vi "test-linear-quadratic-regulator.vi"(8 "error in (no error)":errorcluster) -> (0 "error out":errorcluster, 3 "ALL TESTS GOOD":bool)   [LabVIEW 2019]
uses:
  <vilib>/Rock Robotics/WPI/ThirdParty/JAS_Junk/TrajLib/LINEAR_SYSTEM.ctl
  <vilib>/Analysis/Matrix/Datatypes/RealMatrix.ctl
  <vilib>/Rock Robotics/WPI/ThirdParty/JAS_Junk/TrajLib/LINEAR_QUADRATIC_REGULATOR.ctl
  <vilib>/Rock Robotics/WPI/ThirdParty/JAS_Junk/TrajLib/MatBuilder_Create.vi
  <vilib>/Rock Robotics/WPI/ThirdParty/JAS_Junk/TrajLib/DCMotor_New.vi
  <vilib>/Rock Robotics/WPI/ThirdParty/JAS_Junk/TrajLib/Units_RotationsPerMinuteToRadiansPerSecond.vi
  <vilib>/Rock Robotics/WPI/ThirdParty/JAS_Junk/TrajLib/MatrixHelper_Zero.vi
  <vilib>/Rock Robotics/WPI/ThirdParty/JAS_Junk/TrajLib/LinearSystem_New.vi
  <vilib>/Rock Robotics/WPI/ThirdParty/JAS_Junk/TrajLib/Trajectory_Library.lvlib
  <vilib>/Analysis/Matrix/NI_Matrix.lvlib
panel:
  out "Test 5 Good":bool
  out "Test 4-1 Good":bool
  out "Test 2 Good":bool
  out "Test 1 Good":bool
  out "K 5":T1
  out "Error 5":bool
  out "LinearQuadraticRegulator 5":T2
  out "Relms 5":T1
  out "Qelms 5":T1
  out "ElevatorSystem 5":T3
  out "K 4":T1
  out "ExponentNotRational 4-1":bool
  out "Error 4-1":bool
  out "Error 4":bool
  out "K 4-1":T1
  out "LinearQuadraticRegulator 4":T2
  out "Relms 4":T1
  out "Qelms 4":T1
  out "ElevatorSystem 4":T3
  out "Error 2":bool
  out "K 2":T1
  out "LinearQuadraticRegulator 2":T2
  out "Relms 2":T1
  out "Qelms 2":T1
  out "ElevatorSystem 2":T3
  out "K 1":T1
  out "Error 1":bool
  out "Relms 1":T1
  out "Qelms 1":T1
  out "LQR New Sys-ELMS 1":T2
  out "ElevatorSystem 1":T3
  # "assertEquals(522.153, k.get(0, 0), 0.1);\n    assertEquals(38.2, k.get(0, 1), 0.1);"
  # "assertEquals(10.381, regulator.getK().get(0, 0), 1e-2);\n    assertEquals(0.6929, regulator.getK().get(0, 1), 1e-2);"
  # "assertEquals(8.97115941, regulator.getK().get(0, 0), 1e-3);\n    assertEquals(0.07904881, regulator.getK().get(0, 1), 1e-3);"
  # "assertEquals(19.16, k.get(0, 0), 0.1);\n    assertEquals(3.32, k.get(0, 1), 0.1);"
  # "Ref State <States,1>"
  # "Comp and capped \noutput <Inputs,1>"
  # "Controller gain\n<Inputs,States>"
  # "<States,States>"
  # "<States,Inputs>"
  # "<Outputs,States>"
  # "<Outputs,Inputs>"
  # "Ref State <States,1>"
  # "Comp and capped \noutput <Inputs,1>"
  # "Controller gain\n<Inputs,States>"
  # "<States,States>"
  # "<States,Inputs>"
  # "<Outputs,States>"
  # "<Outputs,Inputs>"
  # "Ref State <States,1>"
  # "Comp and capped \noutput <Inputs,1>"
  # "Controller gain\n<Inputs,States>"
  # "<States,States>"
  # "<States,Inputs>"
  # "<Outputs,States>"
  # "<Outputs,Inputs>"
  # "Ref State <States,1>"
  # "Comp and capped \noutput <Inputs,1>"
  # "Controller gain\n<Inputs,States>"
  # "<States,States>"
  # "<States,Inputs>"
  # "<Outputs,States>"
  # "<Outputs,Inputs>"
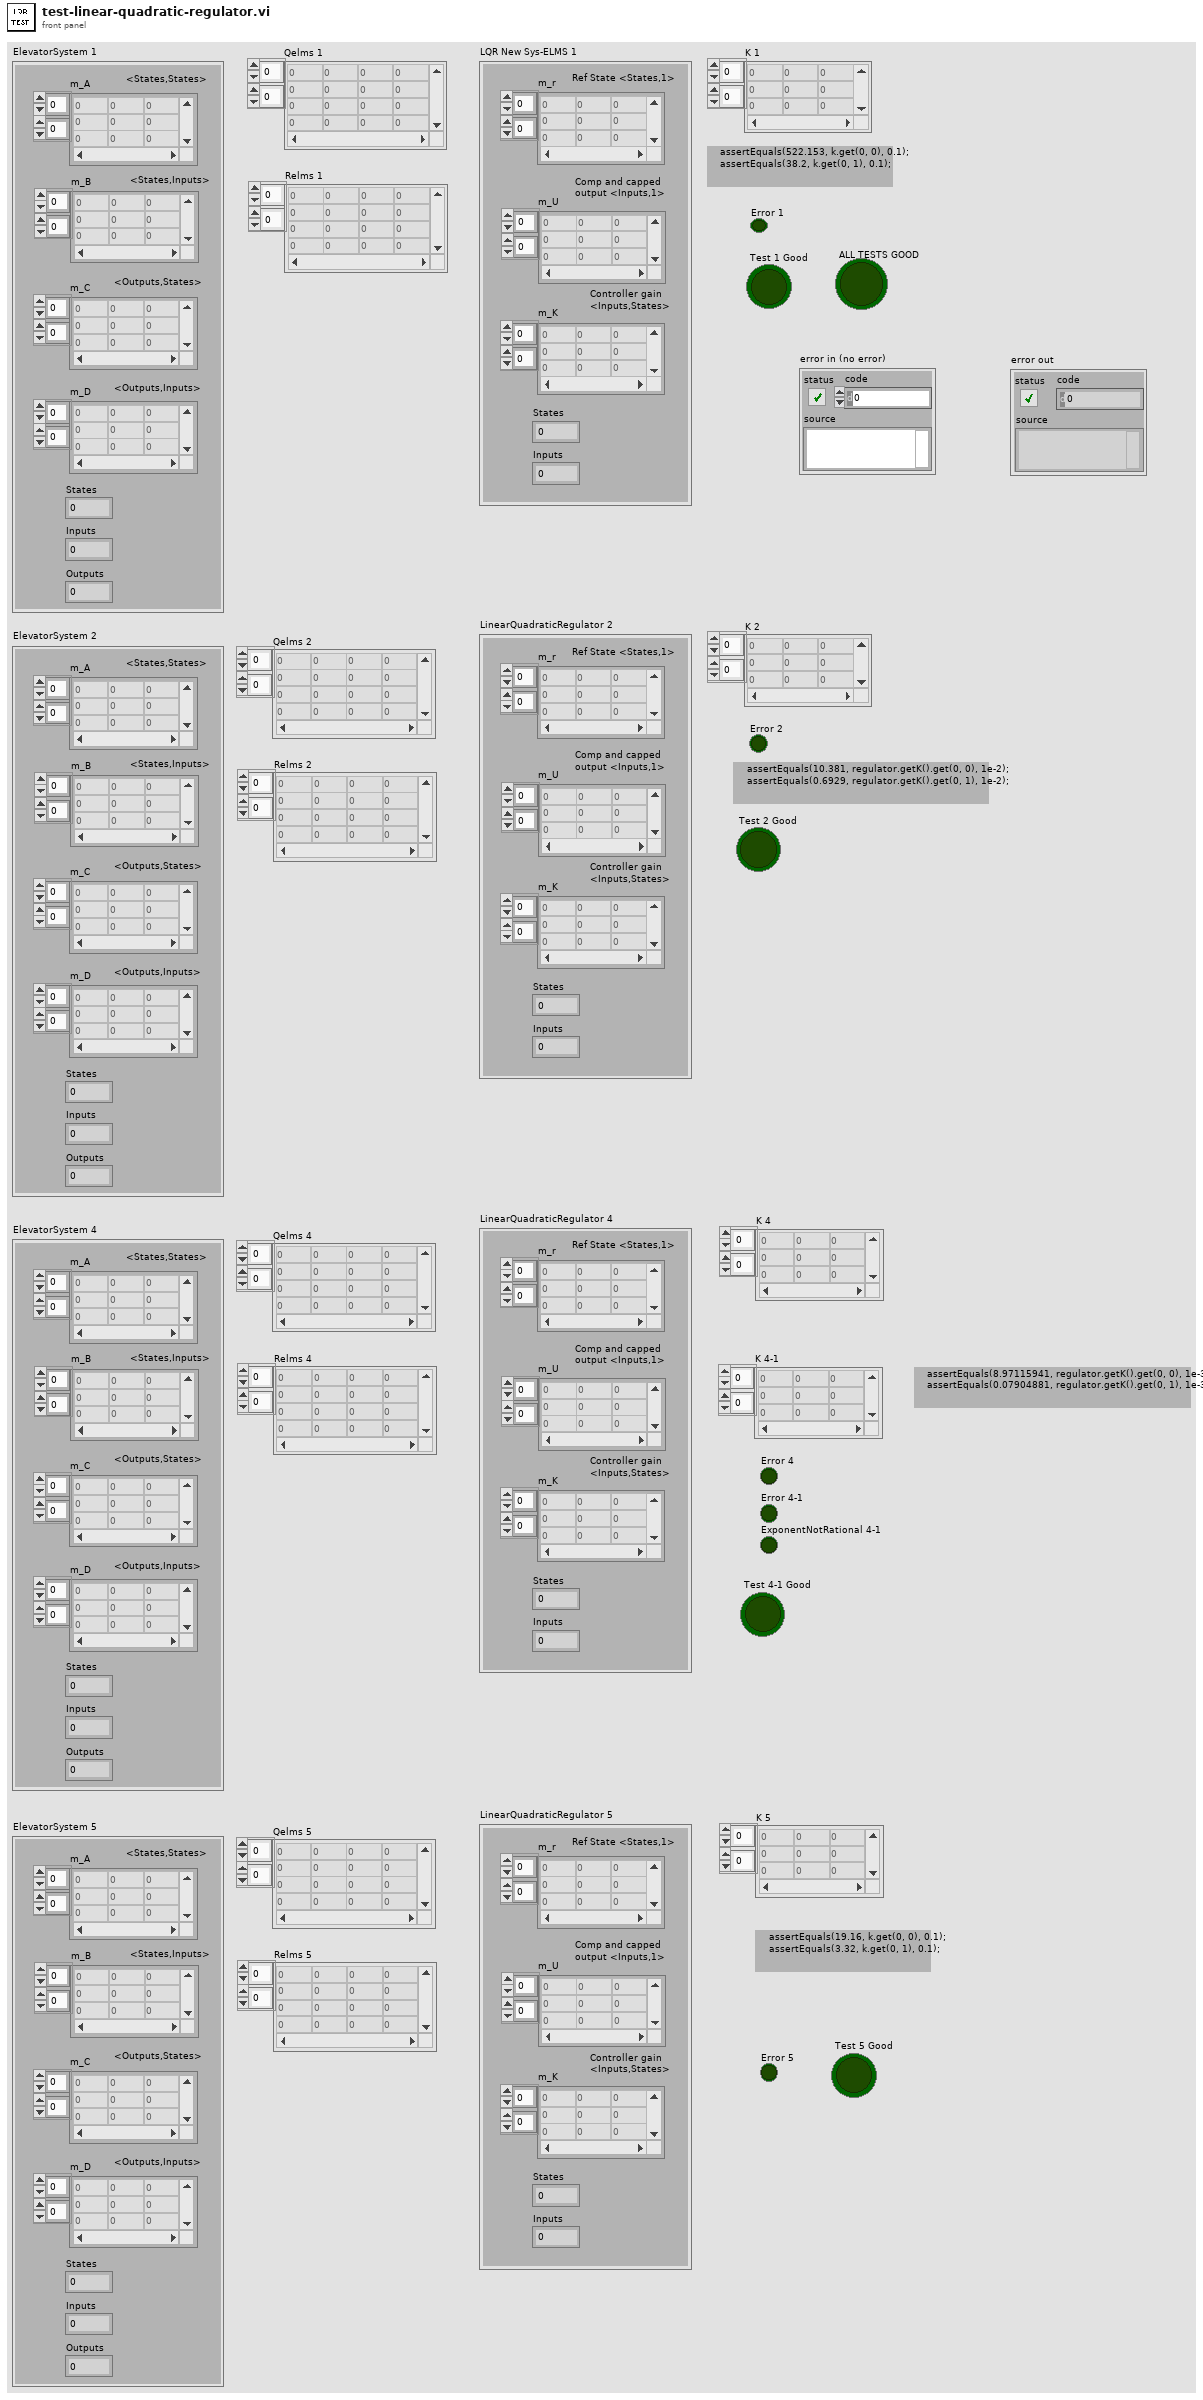
[diagram p1: front panel]
types:
  T1 = typedef "NI_Matrix.lvlib/RealMatrix.ctl" = dbl[][]
  T2 = typedef "Trajectory_Library.lvlib/LINEAR_QUADRATIC_REGULATOR.ctl" = cluster{"m_r":T1, "m_U":T1, "m_K":T1, "States":i32, "Inputs":i32}
  T3 = typedef "Trajectory_Library.lvlib/LINEAR_SYSTEM.ctl" = cluster{"m_A":T1, "m_B":T1, "m_C":T1, "m_D":T1, "States":i32, "Inputs":i32, "Outputs":i32}
  T4 = typedef "Trajectory_Library.lvlib/DCMOTOR.CTL" = cluster{"nominalVoltage_Volts":dbl, "StallTorque_NM":dbl, "StallCurrent_Amps":dbl, "FreeCurrent_Amps":dbl, "FreeSpeed_RadPerSec":dbl, "R_Ohms":dbl, "KvINV_RadPerSecPerVolt":dbl, "Kt_NMPerAmp":dbl, "L_H":dbl, "Jr_KgM2":dbl}
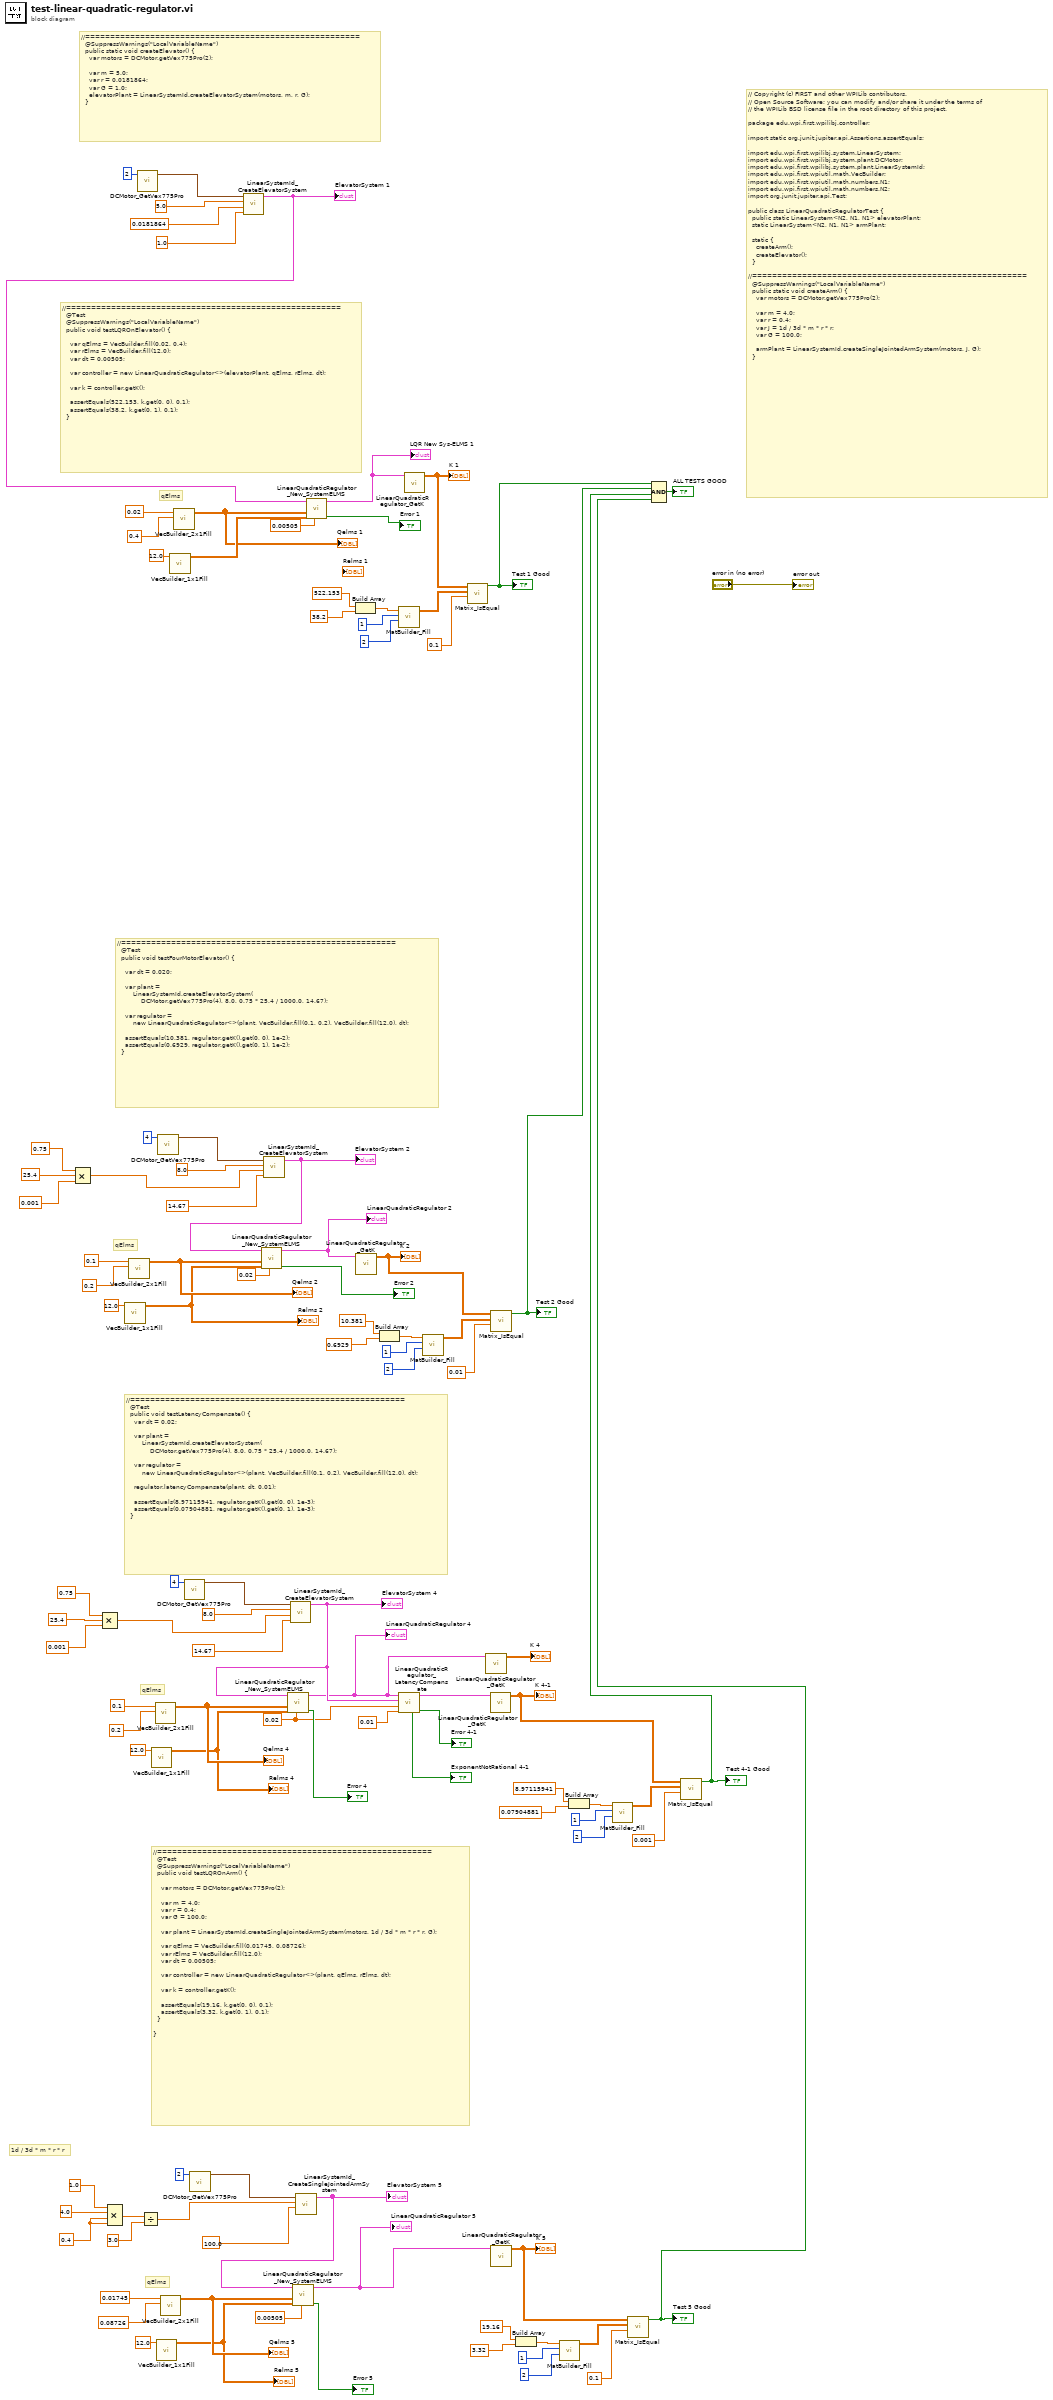
[diagram p0: block diagram]
diagram:
  w43 = 0.4 ("value")
  w63 = 0.02 ("dt_Seconds")
  # "1d / 3d * m * r * r"
  # "qElms"
  # "//=======================================================\n  @Test\n  @SuppressWarnings(\"LocalVariableName\")\n  public void testLQROnArm() {\n\n    var motors = DCMotor.getVex775Pro(2);\n\n    var m = 4.0;\n    var r = 0.4;\n    var G = 100.0;\n\n    var plant = LinearSystemId.createSingleJointedArmSystem(motors, 1d / 3d * m * r * r, G);\n\n    var qElms = VecBuilder.fill(0.01745, 0.08726);\n    var rElms = VecBuilder.fill(12.0);\n    var dt = 0.00505;\n\n    var controller = new LinearQuadraticRegulator<>(plant, qElms, rElms, dt);\n\n    var k = controller.getK();\n\n    assertEquals(19.16, k.get(0, 0), 0.1);\n    assertEquals(3.32, k.get(0, 1), 0.1);\n  }\n\n}"
  # "qElms"
  # "//=======================================================\n  @Test\n  public void testLatencyCompensate() {\n    var dt = 0.02;\n\n    var plant =\n        LinearSystemId.createElevatorSystem(\n            DCMotor.getVex775Pro(4), 8.0, 0.75 * 25.4 / 1000.0, 14.67);\n\n    var regulator =\n        new LinearQuadraticRegulator<>(plant, VecBuilder.fill(0.1, 0.2), VecBuilder.fill(12.0), dt);\n\n    regulator.latencyCompensate(plant, dt, 0.01);\n\n    assertEquals(8.97115941, regulator.getK().get(0, 0), 1e-3);\n    assertEquals(0.07904881, regulator.getK().get(0, 1), 1e-3);\n  }"
  # "qElms"
  # "//=======================================================\n  @Test\n  public void testFourMotorElevator() {\n\n    var dt = 0.020;\n\n    var plant =\n        LinearSystemId.createElevatorSystem(\n            DCMotor.getVex775Pro(4), 8.0, 0.75 * 25.4 / 1000.0, 14.67);\n\n    var regulator =\n        new LinearQuadraticRegulator<>(plant, VecBuilder.fill(0.1, 0.2), VecBuilder.fill(12.0), dt);\n\n    assertEquals(10.381, regulator.getK().get(0, 0), 1e-2);\n    assertEquals(0.6929, regulator.getK().get(0, 1), 1e-2);\n  }"
  # "//=======================================================\n  @SuppressWarnings(\"LocalVariableName\")\n  public static void createElevator() {\n    var motors = DCMotor.getVex775Pro(2);\n\n    var m = 5.0;\n    var r = 0.0181864;\n    var G = 1.0;\n    elevatorPlant = LinearSystemId.createElevatorSystem(motors, m, r, G);\n  }"
  # "qElms"
  # "//=======================================================\n  @Test\n  @SuppressWarnings(\"LocalVariableName\")\n  public void testLQROnElevator() {\n\n    var qElms = VecBuilder.fill(0.02, 0.4);\n    var rElms = VecBuilder.fill(12.0);\n    var dt = 0.00505;\n\n    var controller = new LinearQuadraticRegulator<>(elevatorPlant, qElms, rElms, dt);\n\n    var k = controller.getK();\n\n    assertEquals(522.153, k.get(0, 0), 0.1);\n    assertEquals(38.2, k.get(0, 1), 0.1);\n  }"
  # "// Copyright (c) FIRST and other WPILib contributors.\n// Open Source Software; you can modify and/or share it under the terms of\n// the WPILib BSD license file in the root directory of this project.\n\npackage edu.wpi.first.wpilibj.controller;\n\nimport static org.junit.jupiter.api.Assertions.assertEquals;\n\nimport edu.wpi.first.wpilibj.system.LinearSystem;\nimport edu.wpi.first.wpilibj.system.plant.DCMotor;\nimport edu.wpi.first.wpilibj.system.plant.LinearSystemId;\nimport edu.wpi.first.wpiutil.math.VecBuilder;\nimport edu.wpi.first.wpiutil.math.numbers.N1;\nimport edu.wpi.first.wpiutil.math.numbers.N2;\nimport org.junit.jupiter.api.Test;\n\npublic class LinearQuadraticRegulatorTest {\n  public static LinearSystem<N2, N1, N1> elevatorPlant;\n  static LinearSystem<N2, N1, N1> armPlant;\n\n  static {\n    createArm();\n    createElevator();\n  }\n\n//=======================================================\n  @SuppressWarnings(\"LocalVariableName\")\n  public static void createArm() {\n    var motors = DCMotor.getVex775Pro(2);\n\n    var m = 4.0;\n    var r = 0.4;\n    var J = 1d / 3d * m * r * r;\n    var G = 100.0;\n\n    armPlant = LinearSystemId.createSingleJointedArmSystem(motors, J, G);\n  }"
  n1 = Compound Arithmetic op=MULTIPLY(0.75 ("value"), 25.4 ("value"), 0.001 ("value")) -> (w88:dbl)
  n2 = Compound Arithmetic op=MULTIPLY(0.75 ("value"), 25.4 ("value"), 0.001 ("value")) -> (w71:dbl)
  n3 = Compound Arithmetic op=MULTIPLY(1.0 ("value"), 4.0 ("value"), w43, w43) -> (w42:dbl)
  n4 = call <vilib>:"VecBuilder_1x1Fill.vi"("R0_C0"=12.0) -> ("output matrix"=w81:T1)  [unwired: 10 in]
  "Relms 2" <- w81
  n5 = call <vilib>:"VecBuilder_2x1Fill.vi"("R1"=0.2, "R0"=0.1) -> ("output matrix"=w83:T1)  [unwired: 9 in]
  "Qelms 2" <- w83
  n6 = call <vilib>:"DCMotor_GetVex775Pro.vi"("Num Motors"=2) -> ("DCMOTOR"=w105:T4)  [unwired: 10 in]
  n7 = Divide(x=w42, y=3.0) -> (x/y=w40:dbl)
  n8 = call <vilib>:"VecBuilder_1x1Fill.vi"("R0_C0"=12.0) -> ("output matrix"=w66:T1)  [unwired: 10 in]
  "Relms 4" <- w66
  n9 = call <vilib>:"VecBuilder_2x1Fill.vi"("R1"=0.2, "R0"=0.1) -> ("output matrix"=w67:T1)  [unwired: 9 in]
  "Qelms 4" <- w67
  n10 = call <vilib>:"VecBuilder_1x1Fill.vi"("R0_C0"=12.0) -> ("output matrix"=w48:T1)  [unwired: 10 in]
  "Relms 5" <- w48
  n11 = call <vilib>:"DCMotor_GetVex775Pro.vi"("Num Motors"=4) -> ("DCMOTOR"=w94:T4)  [unwired: 10 in]
  n12 = call <vilib>:"VecBuilder_2x1Fill.vi"("R1"=0.08726, "R0"=0.01745) -> ("output matrix"=w49:T1)  [unwired: 9 in]
  "Qelms 5" <- w49
  n13 = call <vilib>:"VecBuilder_1x1Fill.vi"("R0_C0"=12.0) -> ("output matrix"=w100:T1)  [unwired: 10 in]
  n14 = call <vilib>:"VecBuilder_2x1Fill.vi"("R1"=0.4, "R0"=0.02) -> ("output matrix"=w99:T1)  [unwired: 9 in]
  "Qelms 1" <- w99
  n15 = call <vilib>:"DCMotor_GetVex775Pro.vi"("Num Motors"=4) -> ("DCMOTOR"=w77:T4)  [unwired: 10 in]
  n16 = call <vilib>:"DCMotor_GetVex775Pro.vi"("Num Motors"=2) -> ("DCMOTOR"=w56:T4)  [unwired: 10 in]
  n17 = call <vilib>:"LinearSystemId_CreateElevatorSystem.vi"("G"=1.0, "radiusMeters"=0.0181864, "massKg"=5.0, "DCMOTOR"=w105) -> ("Linearsystem"=w98:T3)  [unwired: 6 in, 1 out]
  "ElevatorSystem 1" <- w98
  n18 = call <vilib>:"LinearSystemId_CreateElevatorSystem.vi"("G"=14.67, "radiusMeters"=w88, "massKg"=8.0, "DCMOTOR"=w94) -> ("Linearsystem"=w82:T3)  [unwired: 6 in, 1 out]
  "ElevatorSystem 2" <- w82
  n19 = call <vilib>:"LinearQuadraticRegulator_New_SystemELMS.vi"("dt_Seconds"=0.02, "Relms"=w81, "Qelms"=w83, "LINEARSYSTEM"=w82) -> ("Error"=→"Error 2":bool, "LinearQuadraticRegulator"=w80:T2)  [unwired: 6 in]
  "LinearQuadraticRegulator 2" <- w80
  n20 = call <vilib>:"LinearSystemId_CreateElevatorSystem.vi"("G"=14.67, "radiusMeters"=w71, "massKg"=8.0, "DCMOTOR"=w77) -> ("Linearsystem"=w64:T3)  [unwired: 6 in, 1 out]
  "ElevatorSystem 4" <- w64
  n21 = call <vilib>:"LinearQuadraticRegulator_New_SystemELMS.vi"("dt_Seconds"=w63, "Relms"=w66, "Qelms"=w67, "LINEARSYSTEM"=w64) -> ("Error"=→"Error 4":bool, "LinearQuadraticRegulator"=w58:T2)  [unwired: 6 in]
  "LinearQuadraticRegulator 4" <- w58
  n22 = call <vilib>:"LinearSystemId_CreateSingleJointedArmSystem.vi"("G"=100.0, "jKgSquaredMeters"=w40, "DCMOTOR"=w56) -> ("Linearsystem"=w46:T3)  [unwired: 7 in, 1 out]
  "ElevatorSystem 5" <- w46
  n23 = call <vilib>:"LinearQuadraticRegulator_New_SystemELMS.vi"("dt_Seconds"=0.00505, "Relms"=w48, "Qelms"=w49, "LINEARSYSTEM"=w46) -> ("Error"=→"Error 5":bool, "LinearQuadraticRegulator"=w44:T2)  [unwired: 6 in]
  "LinearQuadraticRegulator 5" <- w44
  n24 = call <vilib>:"LinearQuadraticRegulator_New_SystemELMS.vi"("dt_Seconds"=0.00505, "Relms"=w100, "Qelms"=w99, "LINEARSYSTEM"=w98) -> ("Error"=→"Error 1":bool, "LinearQuadraticRegulator"=w96:T2)  [unwired: 6 in]
  "LQR New Sys-ELMS 1" <- w96
  n25 = Build Array(522.153 ("element"), 38.2 ("element")) -> (w39:dbl[])
  n26 = call <vilib>:"LinearQuadraticRegulator_GetK.vi"("in LinearQuadraticRegulator"=w80) -> ("K"=w24:T1)  [unwired: 10 in]
  "K 2" <- w24
  n27 = Build Array(10.381 ("element"), 0.6929 ("element")) -> (w31:dbl[])
  n28 = call <vilib>:"MatBuilder_Fill.vi"("Columns"=2, "Rows"=1, "Value List"=w39) -> ("output matrix"=w33:T1)  [unwired: 8 in]
  n29 = call <vilib>:"LinearQuadraticRegulator_LatencyCompensate.vi"("InputDelay_Seconds"=0.01, "dT_Seconds"=w63, "Plant"=w64, "in LinearQuadraticRegulator"=w58) -> ("Error"=→"Error 4-1":bool, "out LinearQuadraticRegulator"=w16:T2, "ExponentNotRational"=→"ExponentNotRational 4-1":bool)  [unwired: 5 in]
  n30 = call <vilib>:"LinearQuadraticRegulator_GetK.vi"("in LinearQuadraticRegulator"=w96) -> ("K"=w34:T1)  [unwired: 10 in]
  "K 1" <- w34
  n31 = call <vilib>:"MatBuilder_Fill.vi"("Columns"=2, "Rows"=1, "Value List"=w31) -> ("output matrix"=w26:T1)  [unwired: 8 in]
  n32 = call <vilib>:"Matrix_IsEqual.vi"("Tolerance"=0.1, "other"=w33, "input matrix"=w34) -> ("Equal"=w6:bool)  [unwired: 8 in]
  "Test 1 Good" <- w6
  n33 = call <vilib>:"LinearQuadraticRegulator_GetK.vi"("in LinearQuadraticRegulator"=w58) -> ("K"=→"K 4":T1)  [unwired: 10 in]
  n34 = call <vilib>:"LinearQuadraticRegulator_GetK.vi"("in LinearQuadraticRegulator"=w16) -> ("K"=w15:T1)  [unwired: 10 in]
  "K 4-1" <- w15
  n35 = call <vilib>:"Matrix_IsEqual.vi"("Tolerance"=0.01, "other"=w26, "input matrix"=w24) -> ("Equal"=w5:bool)  [unwired: 8 in]
  "Test 2 Good" <- w5
  n36 = call <vilib>:"LinearQuadraticRegulator_GetK.vi"("in LinearQuadraticRegulator"=w44) -> ("K"=w7:T1)  [unwired: 10 in]
  "K 5" <- w7
  n37 = Build Array(19.16 ("element"), 3.32 ("element")) -> (w14:dbl[])
  n38 = call <vilib>:"MatBuilder_Fill.vi"("Columns"=2, "Rows"=1, "Value List"=w14) -> ("output matrix"=w9:T1)  [unwired: 8 in]
  n39 = Build Array(8.97115941 ("element"), 0.07904881 ("element")) -> (w23:dbl[])
  n40 = call <vilib>:"MatBuilder_Fill.vi"("Columns"=2, "Rows"=1, "Value List"=w23) -> ("output matrix"=w18:T1)  [unwired: 8 in]
  n41 = call <vilib>:"Matrix_IsEqual.vi"("Tolerance"=0.1, "other"=w9, "input matrix"=w7) -> ("Equal"=w3:bool)  [unwired: 8 in]
  "Test 5 Good" <- w3
  n42 = call <vilib>:"Matrix_IsEqual.vi"("Tolerance"=0.001, "other"=w18, "input matrix"=w15) -> ("Equal"=w4:bool)  [unwired: 8 in]
  "Test 4-1 Good" <- w4
  n43 = Compound Arithmetic op=AND(w6, w5, w4, w3) -> (→"ALL TESTS GOOD":bool)
  "error out" <- "error in (no error)"
